vi "HV_Rampset.vi"(9 "Ramp Up/Down":enum16{"Ramp Down", "Ramp Up"}(ring), 10 "Ramp Rate":string="50") -> (3 "Ramp Output":string)   [LabVIEW 2019]
panel:
  # "- Set ramp up and ramp down rates (V/s) for all channels\n- Choose ramp up or ramp down and enter value"
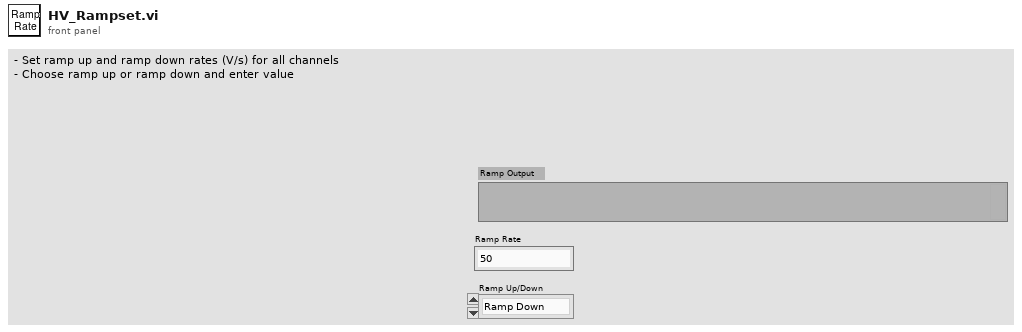
[diagram p1: front panel]
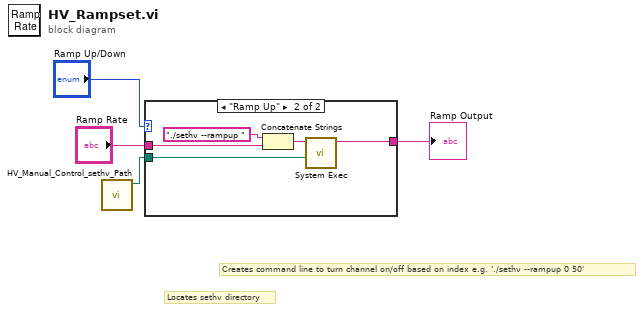
[diagram p0: block diagram]
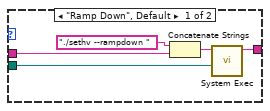
[diagram p2: hidden frame]
diagram:
  # "Locates sethv directory"
  # "Creates command line to turn channel on/off based on index e.g. './sethv --rampup 0 50'"
  n1 = call "HV_Manual_Control_sethv_Path.vi"() -> ("sethv filepath"=w1:path)  [unwired: 11 in]
  n2 = case shown="\"Ramp Up\"" "Ramp Up/Down" {
    tunnel: w1 -> [w6 w11]
    tunnel: "Ramp Rate" -> [w8 w13]
    tunnel: [w5 w10] -> w2
    frame "Ramp Down", Default {
      n3 = Concatenate Strings("./sethv --rampdown " ("command line"), w8) -> (w7:string)
      n4 = call <vilib>:"System Exec.vi"("working directory"=w6, "command line"=w7) -> ("standard output"=w5:string)  [unwired: 6 in, 3 out]
    }
    frame "Ramp Up" {
      n5 = Concatenate Strings("./sethv --rampup " ("command line"), w13) -> (w12:string)
      n6 = call <vilib>:"System Exec.vi"("working directory"=w11, "command line"=w12) -> ("standard output"=w10:string)  [unwired: 6 in, 3 out]
    }
  }
  "Ramp Output" <- w2
